vi "confirm_measured_values_DFA.vi"() -> ()   [LabVIEW 2009]
panel:
  out "last measured value":u16
  in  "LIDAR raw data":u8
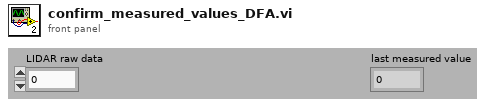
[diagram p1: front panel]
types:
  T1 = enum16{"confirm check sum", "check status byte", "read measured values", "confirm measurement", "confirm command", "read message length", "read address", "wait for \"02\""}
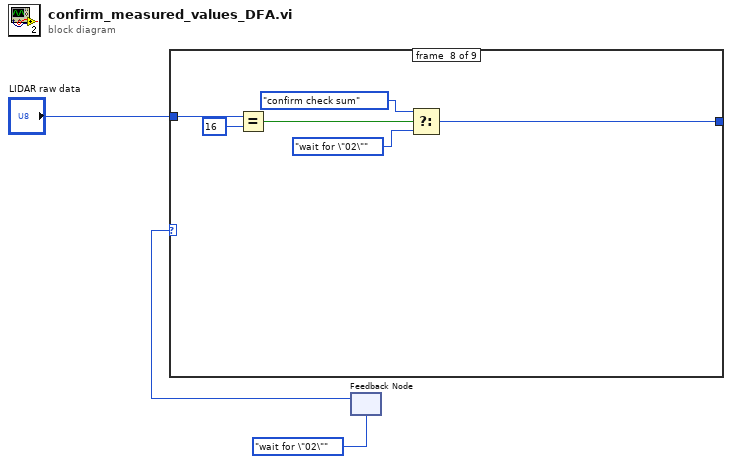
[diagram p0: block diagram]
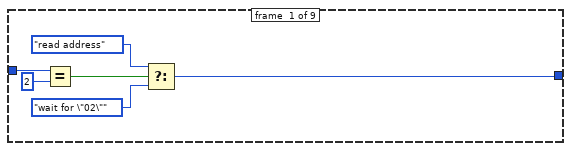
[diagram p2: hidden frame]
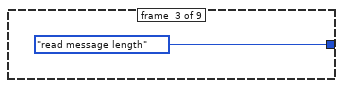
[diagram p4: hidden frame]
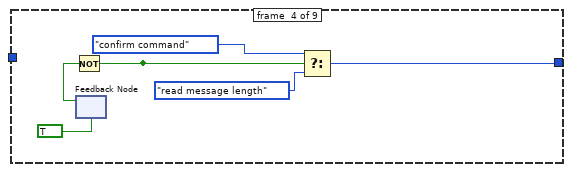
[diagram p5: hidden frame]
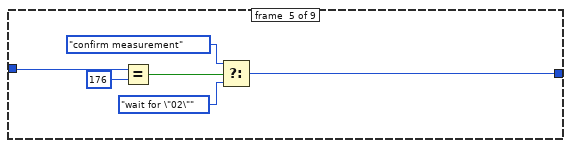
[diagram p6: hidden frame]
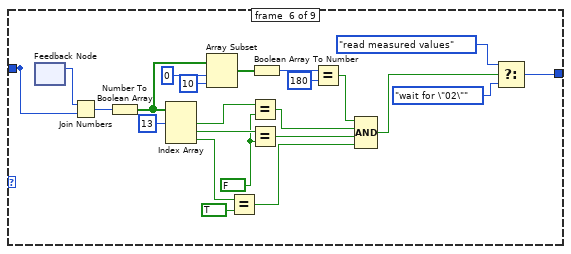
[diagram p7: hidden frame]
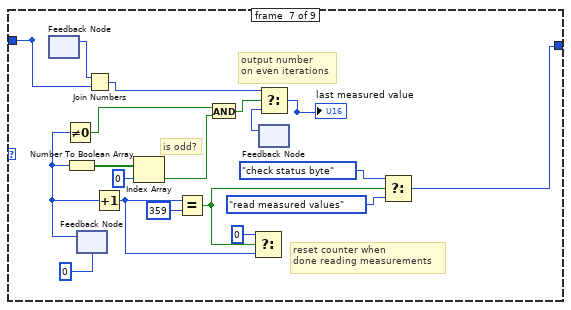
[diagram p8: hidden frame]
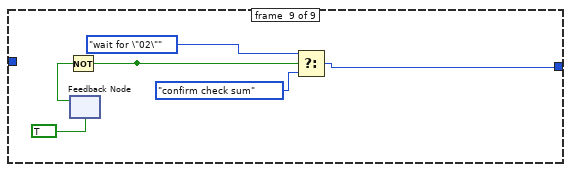
[diagram p9: hidden frame]
diagram:
  n1 = feedback #1(T1."wait for \"02\"") -> (w3:T1)
  n2 = case shown="\"confirm check sum\"" w3 {
    tunnel: "LIDAR raw data" -> [w10 _ _ _ w23 w45 w65 w72 _]
    tunnel: [w5 _ T1."read message length" w13 w18 w27 w48 w67 w73] -> w2
    frame #0 {
      n3 = Equal?(x=w10, y=i8 2) -> (x = y?=w8:bool)
      n4 = Select(t=T1."read address", s=w8, f=T1."wait for \"02\"") -> (s? t:f=w5:T1)
    }
    frame #1 {
    }
    frame #2 {
    }
    frame #3 {
      n5 = feedback #2(TRUE) -> (w17:bool)
      n6 = Not(x=w17) -> (.not. x?=w15:bool)
      n7 = Select(t=T1."confirm command", s=w15, f=T1."read message length") -> (s? t:f=w13:T1)
    }
    frame #4 {
      n8 = Equal?(x=w23, y=u8 176) -> (x = y?=w21:bool)
      n9 = Select(t=T1."confirm measurement", s=w21, f=T1."wait for \"02\"") -> (s? t:f=w18:T1)
    }
    frame #5 {
      w39 = FALSE ("y")
      n10 = feedback #3() -> (w46:u8)  [unwired: 1 in]
      n11 = Join Numbers(hi=w46, lo=w45) -> ((hi.lo)=w44:u16)
      n12 = Number To Boolean Array(number=w44) -> (Boolean array=w34:bool[])
      n13 = Index Array(array=w34, index #1=13 ("index")) -> (element #1=w38:bool, element #2=w40:bool, element #3=w42:bool)  [unwired: 2 in]
      n14 = Array Subset(array=w34, index=0, length=10) -> (w31:bool[])
      n15 = Equal?(x=w42, y=TRUE) -> (x = y?=w35:bool)
      n16 = Equal?(x=w38, y=w39) -> (x = y?=w37:bool)
      n17 = Equal?(x=w40, y=w39) -> (x = y?=w36:bool)
      n18 = Boolean Array To Number(Boolean array=w31) -> (number=w30:u16)
      n19 = Equal?(x=w30, y=u16 180) -> (x = y?=w28:bool)
      n20 = Compound Arithmetic op=AND(w28, w37, w36, w35) -> (w26:bool)
      n21 = Select(t=T1."read measured values", s=w26, f=T1."wait for \"02\"") -> (s? t:f=w27:T1)
    }
    frame #6 {
      # "is odd?"
      # "output number\non even iterations"
      # "reset counter when\ndone reading measurements"
      n22 = feedback #4() -> (w66:u8)  [unwired: 1 in]
      n23 = feedback #5(i16 0) -> (w57:i16)
      n24 = Not Equal To 0?(x=w57) -> (x != 0?=w56:bool)
      n25 = Number To Boolean Array(number=w57) -> (Boolean array=w62:bool[])
      n26 = Join Numbers(hi=w66, lo=w65) -> ((hi.lo)=w60:u16)
      n27 = Increment(x=w57) -> (x+1=w53:i16)
      n28 = Index Array(array=w62, index=0) -> (element=w47:bool)
      n29 = Equal?(x=w53, y=i16 359) -> (x = y?=w51:bool)
      n30 = And(x=w56, y=w47) -> (x .and. y?=w55:bool)
      n31 = Select(t=i16 0, s=w51, f=w53) -> (s? t:f=w54:i16)
      n32 = feedback #6() -> (w58:u16)  [unwired: 1 in]
      n33 = Select(t=w60, s=w55, f=w58) -> (s? t:f=w59:u16)
      "last measured value" <- w59
      n34 = Select(t=T1."check status byte", s=w51, f=T1."read measured values") -> (s? t:f=w48:T1)
    }
    frame #7 {
      n35 = Equal?(x=w72, y=u8 16) -> (x = y?=w70:bool)
      n36 = Select(t=T1."confirm check sum", s=w70, f=T1."wait for \"02\"") -> (s? t:f=w67:T1)
    }
    frame #8 {
      n37 = feedback #7(TRUE) -> (w78:bool)
      n38 = Not(x=w78) -> (.not. x?=w76:bool)
      n39 = Select(t=T1."wait for \"02\"", s=w76, f=T1."confirm check sum") -> (s? t:f=w73:T1)
    }
  }
